vi "init.vi"(8 "error in (no error)":errorcluster, 9 "SG Pin":string, 10 "Measurement Name":string, 11 "Standard":string) -> (0 "error out":errorcluster, 3 "ET_Delay_Sweep out":refnum<class "ET_Delay_Sweep.lvclass">)   [LabVIEW 2016, in "SeqAuto Evaluations.lvlib" / "ET_Delay_Sweep.lvclass"]
uses:
  ET_Delay_Sweep.lvclass
  C:/projects/STS/Common/Sequence Automation/Plugins/SeqAuto IEvaluation.lvlibp/SeqAuto IEvaluation.lvclass
  ET_Delay_Sweep.lvclass/ET_Delay_Sweep.ctl
  Plugins/SeqAuto IEvaluation.lvlibp/Write Measurement Name.vi
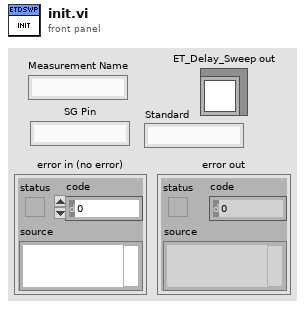
[diagram p1: front panel]
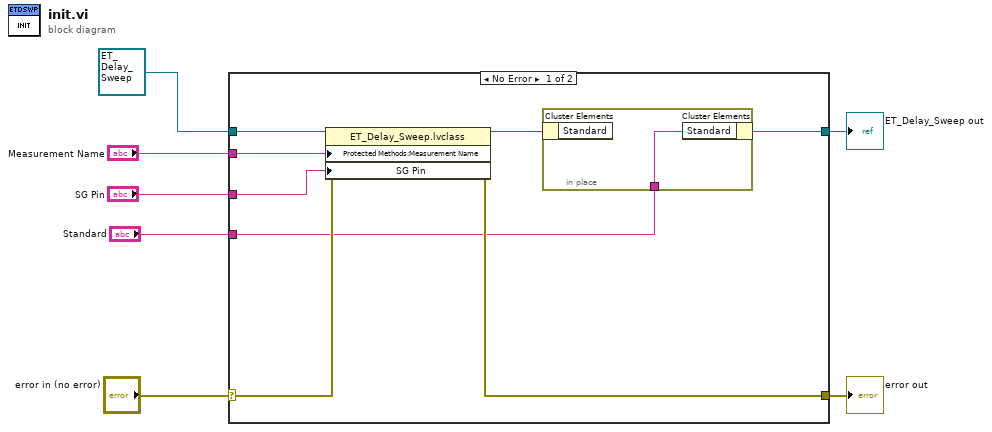
[diagram p0: block diagram]
diagram:
  n1 = case shown="No Error" "error in (no error)" {
    selector: "error in (no error)" -> [w15 w18]
    tunnel: [w14 w18] -> w6
    tunnel: [w9 w17] -> w4
    tunnel: refnum<class "ET_Delay_Sweep.lvclass"> refnum ("ET_Delay_Sweep in") -> [w13 w17]
    tunnel: "Measurement Name" -> [w12 _]
    tunnel: "SG Pin" -> [w11 _]
    tunnel: "Standard" -> [w8 _]
    frame No Error {
      n2 = property class="ET_Delay_Sweep.lvclass"(reference=w13, error in=w15, "Protected Methods:Measurement Name"=w12, "SG Pin"=w11) -> (reference out=w10:refnum<class "ET_Delay_Sweep.lvclass">, error out=w14:errorcluster)
      n3 = in-place {
        in-place-border: w8 -> [w16]
        n4 = in-place-cluster #1(w10) -> ()  [unwired: 1 out]
        n5 = in-place-cluster #1("Standard"=w16) -> (w9:refnum<class "ET_Delay_Sweep.lvclass">)
      }
    }
    frame Error {
    }
  }
  "error out" <- w6
  "ET_Delay_Sweep out" <- w4
